vi "Read Websocket Server Message Transport.vi"(11 "Websocket Message Broker Interface Ref in":refnum<class "Websocket Message Broker Interface Ref.lvclass">) -> (2 "Stream Mediator.lvlib:Message Transport Queue.lvclass":refnum<class "Message Transport Queue.lvclass">, 3 "Websocket Message Broker Interface Ref out":refnum<class "Websocket Message Broker Interface Ref.lvclass">)   [LabVIEW 2016, in "Stream Mediator.lvlib" / "Websocket Message Broker Interface Ref.lvclass"]
uses:
  <userlib>/Composed Systems/Stream/Mediator/Classes/Websocket Message Broker Interface Ref/Websocket Message Broker Interface Ref.lvclass
  <userlib>/Composed Systems/Stream/Mediator/Classes/Message Transport Queue/Message Transport Queue.lvclass
  <userlib>/Composed Systems/Stream/Mediator/Classes/Websocket Message Broker Interface Ref/Websocket Message Broker Interface Ref.lvclass/Websocket Message Broker Interface Ref.ctl
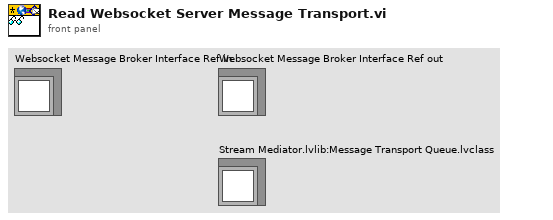
[diagram p1: front panel]
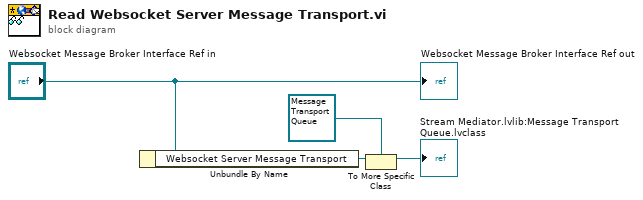
[diagram p0: block diagram]
diagram:
  n1 = Unbundle By Name("Websocket Message Broker Interface Ref in") -> ("Websocket Server Message Transport"=w3:refnum<class "Message Transport Interface.lvclass">)
  n2 = To More Specific Class(target class=refnum<class "Message Transport Queue.lvclass"> refnum ("Stream Mediator.lvlib:Message Transport Queue.lvclass"), reference=w3) -> (specific class reference=→"Stream Mediator.lvlib:Message Transport Queue.lvclass":refnum<class "Message Transport Queue.lvclass">)  [unwired: 1 in, 1 out]
  "Websocket Message Broker Interface Ref out" <- "Websocket Message Broker Interface Ref in"
